vi "UHR-Fleezers Control (host) - 11.9b.vi"() -> ()   [LabVIEW 2014] (continued)
                  n310 = And(x=w552, y=w549) -> (x .and. y?=w551:bool)
                  n311 = case "Only if were fishing and now formed tether" shown="True" w551 {
                    tunnel: w550 -> [w554 w569]
                    tunnel: [w553 w568] -> w548
                    tunnel: w547 -> [_ w564]
                    frame False {
                      n312 = local read "Fish"() -> (w553:bool)
                      n313 = case shown="False" w553 {
                        tunnel: w554 -> [w555 _]
                        frame False {
                          n314 = property on="BD 1 Frequency 1 (MHz)" class="DigNum (strict)"("Val(Sgnl)"=w555) -> ()  [unwired: 2 in, 2 out]
                        }
                        frame True {
                        }
                      }
                    }
                    frame True {
                      w568 = FALSE ("Fish for Tether")
                      n315 = call <vilib>:"Beep.vi"() -> ()  [unwired: 3 in, 9 out]
                      n316 = Number To Decimal String(number=w564, width (-)=i16 1) -> (decimal integer string=w562:string)
                      n317 = Concatenate Strings("Formed tether in ", w562, " attempt(s)." ("string")) -> (w559:string)
                      n318 = local read "Messages"() -> (w566:string)
                      n319 = local write "Fish"(w568) -> ()
                      n320 = call "Update messages.vi"("Message to add"=w559, "Old message string"=w566) -> ("New message string"=w565:string)
                      n321 = local write "Messages"(w565) -> ()
                      n322 = Get Date/Time In Seconds() -> (seconds since 1Jan1904=→"Time tether formed":timestamp)
                      n323 = local read "Flow ON\nduring cal?"() -> (w556:bool)
                      n324 = property on="Sample Channel\nFlow" class="Bool (strict)"("Val(Sgnl)"=w556) -> (error out=w557:errorcluster)  [unwired: 2 in, 1 out]
                      n325 = case shown="\"2\", \"3\", \"4\", \"5\", \"6\"" "Then..." {
                        selector: "Then..." -> [_ w572 _ _]
                        tunnel: w569 -> [w571 _ _ _]
                        tunnel: w557 -> [_ _ _ _]
                        frame "1", Default {
                          n326 = property on="BD 1 Frequency 1 (MHz)" class="DigNum (strict)"("Val(Sgnl)"=w571) -> ()  [unwired: 2 in, 2 out]
                        }
                        frame "2", "3", "4", "5", "6" {
                          n327 = flat-sequence {
                            tunnel: w572 -> [w578]
                            frame #0 {
                              n328 = local read "Flow ON\nduring cal?"() -> (w573:bool)
                              n329 = property on="Sample Channel\nFlow" class="Bool (strict)"("Val(Sgnl)"=w573) -> ()  [unwired: 2 in, 2 out]
                              n330 = property on="Trap D (MHz)" class="DigNum (strict)"("Val(Sgnl)"="Move to D 1 (MHz)") -> ()  [unwired: 2 in, 2 out]
                            }
                            frame #1 {
                              n331 = local read "Wait Before Save (s)"() -> (w575:u32)
                              n332 = Multiply(x=u32 1000 ("milliseconds to wait"), y=w575) -> (x*y=w577:u32)
                              n333 = Wait (ms)(milliseconds to wait=w577) -> ()  [unwired: 1 out]
                            }
                            frame #2 {
                              n334 = case shown="\"5\", \"6\"" w578 {
                                selector: w578 -> [w581 w591 _]
                                frame "3", "4" {
                                n335 = flat-sequence {
                                tunnel: w581 -> [w582]
                                tunnel: [w582] -> w579
                                tunnel: [w584] -> w580
                                tunnel: w579 -> [w584]
                                tunnel: w580 -> [w588]
                                frame #0 {
                                n336 = property on="Green ON/Interlacing" class="Bool (strict)"("Val(Sgnl)"=TRUE ("Value (Signaling)")) -> ()  [unwired: 2 in, 2 out]
                                }
                                frame #1 {
                                n337 = Multiply(x="Wait Before Save (s)", y=u32 1000 ("x")) -> (x*y=w586:u32)
                                n338 = Wait (ms)(milliseconds to wait=w586) -> ()  [unwired: 1 out]
                                }
                                frame #2 {
                                n339 = property on="Start Saving" class="Bool (strict)"("Value"=TRUE ("Start Saving")) -> ()  [unwired: 2 in, 2 out]
                                n340 = case shown="\"4\"" w588 {
                                frame Default {
                                }
                                frame "4" {
                                n341 = property on="Fl. Triggered..." class="Bool (strict)"("Val(Sgnl)"=TRUE ("Value (Signaling)")) -> ()  [unwired: 2 in, 2 out]
                                }
                                }
                                }
                                }
                                }
                                frame "5", "6" {
                                n342 = stacked-sequence {
                                tunnel: w591 -> [_ _ _ _ _ _ w603]
                                frame #0 {
                                n343 = Replace Array Subset(array=u32[] [0] ("Index Values"), new element="Raster Set\nUpon Tether", index=0) -> (w592:u32[])
                                n344 = property on="Saved AOD Raster Scan Parameter Sets" class="Arr (strict)"("Index Values"=w592) -> ()  [unwired: 2 in, 2 out]
                                }
                                frame #1 {
                                n345 = Wait (ms)(milliseconds to wait=u32 500) -> ()  [unwired: 1 out]
                                }
                                frame #2 {
                                n346 = property on="Load parameters" class="Bool (strict)"("Val(Sgnl)"=TRUE ("Value (Signaling)")) -> ()  [unwired: 2 in, 2 out]
                                n347 = case shown="True" "Green ON during\nraster?" {
                                frame False {
                                }
                                frame True {
                                n348 = property on="Green ON/Interlacing" class="Bool (strict)"("Val(Sgnl)"=TRUE ("Value (Signaling)")) -> ()  [unwired: 2 in, 2 out]
                                }
                                }
                                }
                                frame #3 {
                                n349 = Wait (ms)(milliseconds to wait=u32 500) -> ()  [unwired: 1 out]
                                }
                                frame #4 {
                                n350 = property on="Trap Raster Scan" class="Bool (strict)"("Val(Sgnl)"=TRUE ("Value (Signaling)")) -> ()  [unwired: 2 in, 2 out]
                                }
                                frame #5 {
                                n351 = Wait (ms)(milliseconds to wait=u32 2000) -> ()  [unwired: 1 out]
                                }
                                frame #6 {
                                n352 = flat-sequence {
                                tunnel: w603 -> [w610]
                                frame #0 {
                                n353 = while {
                                stop <- w606 stop-if-true
                                n354 = local read "Raster Scanning..."() -> (w605:bool)
                                n355 = local read "Saving..."() -> (w608:bool)
                                n356 = Wait (ms)(milliseconds to wait=u32 100) -> ()  [unwired: 1 out]
                                n357 = Not(x=w608) -> (.not. x?=w607:bool)
                                n358 = Not(x=w605) -> (.not. x?=w604:bool)
                                n359 = And(x=w607, y=w604) -> (x .and. y?=w606:bool)
                                }
                                }
                                frame #1 {
                                n360 = local read "Tether"() -> (w611:bool)
                                n361 = case shown="True" w611 {
                                tunnel: w610 -> [_ w613]
                                frame False {
                                n362 = property on="Fish" class="Bool (strict)"("Val(Sgnl)"="Fish again after \nraster break?") -> ()  [unwired: 2 in, 2 out]
                                }
                                frame True {
                                n363 = stacked-sequence {
                                tunnel: w613 -> [_ w617 _ _ _ _ _ _]
                                frame #0 {
                                n364 = property on="Trap D (MHz)" class="DigNum (strict)"("Val(Sgnl)"="Move to D 2 (MHz)") -> ()  [unwired: 2 in, 2 out]
                                n365 = case shown="True" "Flow ON after\ntether testing?" {
                                frame False {
                                }
                                frame True {
                                n366 = property on="Sample Channel\nFlow" class="Bool (strict)"("Val(Sgnl)"=TRUE ("Value (Signaling)")) -> ()  [unwired: 2 in, 2 out]
                                }
                                }
                                }
                                frame #1 {
                                n367 = flat-sequence {
                                tunnel: w617 -> [w618]
                                frame #0 {
                                n368 = case shown="\"6\"" w618 {
                                frame Default {
                                }
                                frame "6" {
                                n369 = flat-sequence {
                                frame #0 {
                                n370 = Wait (ms)(milliseconds to wait=u32 500) -> ()  [unwired: 1 out]
                                }
                                frame #1 {
                                n371 = property on="Green ON/Interlacing" class="Bool (strict)"("Val(Sgnl)"=TRUE ("Green Laser ON/Interlacing")) -> ()  [unwired: 2 in, 2 out]
                                }
                                }
                                }
                                }
                                }
                                frame #1 {
                                n372 = case shown="True" "Save at end (5, 6)" {
                                selector: "Save at end (5, 6)" -> [_ w622]
                                frame False {
                                }
                                frame True {
                                n373 = flat-sequence {
                                tunnel: w622 -> [w624]
                                frame #0 {
                                n374 = Wait (ms)(milliseconds to wait=u32 500) -> ()  [unwired: 1 out]
                                }
                                frame #1 {
                                n375 = local write "Start Saving"(w624) -> ()
                                }
                                }
                                }
                                }
                                }
                                }
                                }
                                frame #2 {
                                n376 = local read "Bead Sep. Int. Time (s)"() -> (w627:dbl)
                                n377 = Multiply(x=w627, y=1000.0) -> (x*y=w626:dbl)
                                n378 = Wait (ms)(milliseconds to wait=w626) -> ()  [unwired: 1 out]
                                }
                                frame #3 {
                                n379 = property on="Remove Offset" class="Bool (strict)"("Val(Sgnl)"=TRUE ("Value (Signaling)")) -> ()  [unwired: 2 in, 2 out]
                                }
                                frame #4 {
                                n380 = property on="Read FX file" class="Bool (strict)"("Val(Sgnl)"=TRUE ("Value (Signaling)")) -> ()  [unwired: 2 in, 2 out]
                                }
                                frame #5 {
                                n381 = Wait (ms)(milliseconds to wait=u32 300) -> ()  [unwired: 1 out]
                                }
                                frame #6 {
                                n382 = local read "Bad fit error"() -> (w636:dbl)
                                n383 = local read "Fit offset"() -> (w639:dbl)
                                n384 = Greater Or Equal?(x=w636, y="Bad fit thresh") -> (x >= y?=→"Bad fit":bool)
                                n385 = Greater Or Equal?(x=w639, y="Fit offset thresh") -> (x >= y?=→"Multiple tether":bool)
                                n386 = local read "Hyst. error"() -> (w633:dbl)
                                n387 = Greater Or Equal?(x=w633, y="Hysteresis thresh") -> (x >= y?=→"Hysteresis":bool)
                                }
                                frame #7 {
                                w644 = 0
                                n388 = local read "Bad fit error"() -> (w646:dbl)
                                n389 = local read "Hyst. error"() -> (w645:dbl)
                                n390 = local read "Fit offset"() -> (w647:dbl)
                                n391 = local read "Multiple tether"() -> (w653:bool)
                                n392 = local read "Hysteresis"() -> (w651:bool)
                                n393 = local read "Bad fit"() -> (w652:bool)
                                n394 = Not(x=w651) -> (.not. x?=w643:bool)
                                n395 = Not(x=w652) -> (.not. x?=w649:bool)
                                n396 = Greater?(x=w647, y=w644) -> (0:w642:bool)
                                n397 = Greater?(x=w646, y=w644) -> (0:w641:bool)
                                n398 = Greater?(x=w645, y=w644) -> (0:w640:bool)
                                n399 = Not(x=w653) -> (.not. x?=w650:bool)
                                n400 = Compound Arithmetic op=AND(w650, w649, w643, w642, w641, w640) -> (w648:bool)
                                "Good tether" <- w648
                                n401 = case shown="True" w648 {
                                frame False {
                                }
                                frame True {
                                n402 = call <vilib>:"Beep.vi"("use system alert? (T)"=FALSE, "duration (msec)"=u32 200, "frequency (Hz)"=u32 2000) -> ()  [unwired: 9 in]
                                }
                                }
                                }
                                }
                                }
                                }
                                }
                                }
                                }
                                }
                                }
                                frame "2", Default {
                                }
                              }
                            }
                            frame #3 {
                              n403 = local read "Multiple tether"() -> (w659:bool)
                              n404 = And(x="Break multiple", y=w659) -> (x .and. y?=w657:bool)
                              n405 = case shown="True" w657 {
                                frame False {
                                }
                                frame True {
                                n406 = stacked-sequence {
                                frame #0 {
                                n407 = property on="Trap D (MHz)" class="DigNum (strict)"("Val(Sgnl)"="Trap D to \nbreak (MHz)") -> ()  [unwired: 2 in, 2 out]
                                }
                                frame #1 {
                                n408 = case shown="True" "Fish after\nmultiple break" {
                                frame False {
                                }
                                frame True {
                                n409 = while {
                                stop <- w664 stop-if-true
                                n410 = local read "Multiple tether"() -> (w666:bool)
                                n411 = local read "Fish"() -> (w663:bool)
                                n412 = local read "Stop All"() -> (w662:bool)
                                n413 = Wait (ms)(milliseconds to wait=u32 100) -> ()  [unwired: 1 out]
                                n414 = Not(x=w666) -> (.not. x?=w665:bool)
                                n415 = Compound Arithmetic op=OR(w662, w665, w663) -> (w664:bool)
                                }
                                }
                                }
                                }
                                frame #2 {
                                n416 = local read "Fish after\nmultiple break"() -> (w671:bool)
                                n417 = local read "Stage Moving"() -> (w670:bool)
                                n418 = Not(x=w670) -> (.not. x?=w668:bool)
                                n419 = And(x=w671, y=w668) -> (x .and. y?=w669:bool)
                                n420 = property on="Fish" class="Bool (strict)"("Val(Sgnl)"=w669) -> ()  [unwired: 2 in, 2 out]
                                }
                                }
                                }
                              }
                            }
                            frame #4 {
                              n421 = local read "Bad fit"() -> (w673:bool)
                              n422 = And(x="Break bad fit", y=w673) -> (x .and. y?=w672:bool)
                              n423 = case shown="True" w672 {
                                frame False {
                                }
                                frame True {
                                n424 = stacked-sequence {
                                frame #0 {
                                n425 = local read "Trap D to \nbreak (MHz)"() -> (w675:dbl)
                                n426 = property on="Trap D (MHz)" class="DigNum (strict)"("Val(Sgnl)"=w675) -> ()  [unwired: 2 in, 2 out]
                                }
                                frame #1 {
                                n427 = case shown="True" "Fish after\nbad fit break?" {
                                frame False {
                                }
                                frame True {
                                n428 = while {
                                stop <- w679 stop-if-true
                                n429 = local read "Stop All"() -> (w677:bool)
                                n430 = local read "Bad fit"() -> (w678:bool)
                                n431 = local read "Fish"() -> (w680:bool)
                                n432 = Not(x=w678) -> (.not. x?=w681:bool)
                                n433 = Wait (ms)(milliseconds to wait=u32 100) -> ()  [unwired: 1 out]
                                n434 = Compound Arithmetic op=OR(w677, w681, w680) -> (w679:bool)
                                }
                                }
                                }
                                }
                                frame #2 {
                                n435 = local read "Fish after\nbad fit break?"() -> (w683:bool)
                                n436 = local read "Stage Moving"() -> (w686:bool)
                                n437 = Not(x=w686) -> (.not. x?=w685:bool)
                                n438 = And(x=w683, y=w685) -> (x .and. y?=w684:bool)
                                n439 = property on="Fish" class="Bool (strict)"("Val(Sgnl)"=w684) -> ()  [unwired: 2 in, 2 out]
                                }
                                }
                                }
                              }
                            }
                            frame #5 {
                              n440 = local read "Hysteresis"() -> (w688:bool)
                              n441 = And(x="Break hyst", y=w688) -> (x .and. y?=w687:bool)
                              n442 = case shown="True" w687 {
                                frame False {
                                }
                                frame True {
                                n443 = stacked-sequence {
                                frame #0 {
                                n444 = local read "Trap D to \nbreak (MHz)"() -> (w690:dbl)
                                n445 = property on="Trap D (MHz)" class="DigNum (strict)"("Val(Sgnl)"=w690) -> ()  [unwired: 2 in, 2 out]
                                }
                                frame #1 {
                                n446 = case shown="True" "Fish ater hyst?" {
                                frame False {
                                }
                                frame True {
                                n447 = while {
                                stop <- w696 stop-if-true
                                n448 = local read "Hysteresis"() -> (w695:bool)
                                n449 = local read "Stop All"() -> (w692:bool)
                                n450 = local read "Fish"() -> (w693:bool)
                                n451 = Wait (ms)(milliseconds to wait=u32 100) -> ()  [unwired: 1 out]
                                n452 = Not(x=w695) -> (.not. x?=w694:bool)
                                n453 = Compound Arithmetic op=OR(w692, w694, w693) -> (w696:bool)
                                }
                                }
                                }
                                }
                                frame #2 {
                                n454 = local read "Fish ater hyst?"() -> (w701:bool)
                                n455 = local read "Stage Moving"() -> (w700:bool)
                                n456 = Not(x=w700) -> (.not. x?=w699:bool)
                                n457 = And(x=w701, y=w699) -> (x .and. y?=w698:bool)
                                n458 = property on="Fish" class="Bool (strict)"("Val(Sgnl)"=w698) -> ()  [unwired: 2 in, 2 out]
                                }
                                }
                                }
                              }
                            }
                            frame #6 {
                              n459 = local read "Good tether"() -> (w702:bool)
                              n460 = case shown="True" w702 {
                                frame False {
                                }
                                frame True {
                                n461 = case shown="\"1\"" "If good, then:" {
                                frame "0", Default {
                                }
                                frame "1" {
                                n462 = property on="Force FB Script" class="Bool (strict)"("Val(Sgnl)"=TRUE ("Value (Signaling)")) -> ()  [unwired: 2 in, 2 out]
                                }
                                }
                                }
                              }
                            }
                          }
                        }
                        frame "7" {
                          n463 = property on="Force FB Script" class="Bool (strict)"("Val(Sgnl)"=TRUE ("Value (Signaling)")) -> ()  [unwired: 2 in, 2 out]
                        }
                        frame "8" {
                          n464 = property on="Fixed Traps Script" class="Bool (strict)"("Val(Sgnl)"=TRUE ("Value (Signaling)")) -> ()  [unwired: 2 in, 2 out]
                        }
                      }
                      "Tether" <- "Tether Alarm?"
                    }
                  }
                }
                frame #2 {
                  n465 = local read "Oscillate Set 1"() -> (w712:bool)
                  n466 = local read "Stop All"() -> (w710:bool)
                  n467 = Or(x=w712, y=w707) -> (x .or. y?=w709:bool)
                  n468 = Not(x=w709) -> (.not. x?=w711:bool)
                  n469 = Compound Arithmetic op=OR(w710, w711) -> (w708:bool)
                }
              }
              n470 = node-c288() -> ()  [unwired: 2 out]
            }
            n471 = node-c288(w462) -> ()  [unwired: 1 out]
          }
        }
      }
      event "Fl. Triggered...": Value Change {
        n472 = event-data() -> ()  [unwired: 7 out]
        n473 = case shown="True" "Fl. Triggered..." {
          frame False {
          }
          frame True {
            n474 = node-c288() -> (w723:T21)  [unwired: 4 out]
            n475 = timed-loop {
              timing: w723 -> [_]
              timing-out: [_] -> w722
              tunnel: "Action" -> [w731]
              shift-right: [w728] -> _
              shift-left: u8 255 -> [w730]
              shift-right: [w725] -> _
              shift-left: 255 -> [w727]
              stop <- w724 stop-if-true
              # "Reset confocal spot"
              n476 = node-c288() -> ()  [unwired: 2 out]
              n477 = flat-sequence {
                tunnel: w731 -> [w751]
                tunnel: w730 -> [w750]
                tunnel: [w749] -> w729
                tunnel: w727 -> [w736]
                tunnel: [w735] -> w726
                tunnel: [w1135] -> w724
                tunnel: w729 -> [w1134]
                tunnel: [w1134] -> w728
                tunnel: [w1133] -> w725
                tunnel: w726 -> [w1133]
                frame #0 {
                  n478 = local read "Delta Fl. 2"() -> (w748:dbl)
                  n479 = local read "Delta Fl. 1"() -> (w743:dbl)
                  n480 = Multiply(x="Fl. D Thresh. (kHz)", y=1000.0) -> (x*y=w738:dbl)
                  n481 = Select(t=w743, s="APD to Watch", f=w748) -> (s? t:f=w739:dbl)
                  n482 = Greater?(x=w739, y=w738) -> (0:w744:bool)
                  n483 = Or(x="Force Yank", y=w744) -> (x .or. y?=w742:bool)
                  n484 = And(x=w742, y="Yank when?") -> (x .and. y?=w740:bool)
                  n485 = case shown="False" w740 {
                    tunnel: w751 -> [w754 w957]
                    tunnel: w750 -> [w756 w953]
                    tunnel: [w756 w951] -> w749
                    tunnel: w739 -> [w762 _]
                    tunnel: w738 -> [w761 _]
                    tunnel: "Force Yank" -> [w759 _]
                    tunnel: w736 -> [w758 w950]
                    tunnel: [w757 w950] -> w735
                    frame False {
                      n486 = Negate(x=w761) -> (-x=w753:dbl)
                      n487 = local write "Fl. High"(TRUE ("Fl. High")) -> ()
                      n488 = Less?(x=w762, y=w753) -> (x < y?=w760:bool)
                      n489 = Or(x=w759, y=w760) -> (x .or. y?=w755:bool)
                      n490 = case shown="True" w755 {
                        tunnel: w758 -> [w763 w773]
                        tunnel: [w763 w772] -> w757
                        tunnel: w754 -> [_ w771]
                        frame False {
                        }
                        frame True {
                          n491 = flat-sequence {
                            tunnel: w773 -> [w779]
                            tunnel: w771 -> [w776]
                            tunnel: [w778] -> w770
                            tunnel: [w777] -> w769
                            tunnel: [w776] -> w768
                            tunnel: w767 -> [w775]
                            tunnel: [w775] -> w766
                            tunnel: w765 -> [w774]
                            tunnel: [w774] -> w764
                            tunnel: [w851] -> w772
                            tunnel: w770 -> [w851]
                            tunnel: w769 -> [w850]
                            tunnel: w768 -> [w849]
                            tunnel: w766 -> [w848]
                            tunnel: w764 -> [w847]
                            frame #0 {
                              n492 = call <vilib>:"Beep.vi"() -> ()  [unwired: 12 in]
                              n493 = local write "Waiting"(FALSE ("Waiting")) -> ()
                              n494 = Increment(x=w779) -> (x+1=w778:i32)
                              n495 = case shown="\"Yank\"" w776 {
                                tunnel: w778 -> [_ w784 _]
                                frame "Alarm", Default {
                                }
                                frame "Yank" {
                                n496 = flat-sequence {
                                tunnel: w784 -> [w787]
                                tunnel: [w786] -> w783
                                tunnel: [w785] -> w782
                                tunnel: w783 -> [w797]
                                tunnel: w782 -> [w798]
                                frame #0 {
                                n497 = local read "Yank Delay (s)"() -> (w790:dbl)
                                n498 = local read "N Array El"() -> (w785:u8)
                                n499 = Quotient & Remainder(x=w787, y=w785) -> (x-y*floor(x/y)=w786:i32)  [unwired: 1 out]
                                n500 = Multiply(x=w790, y=1000.0) -> (x*y=w788:dbl)
                                n501 = Wait (ms)(milliseconds to wait=w788) -> ()  [unwired: 1 out]
                                }
                                frame #1 {
                                n502 = local read "Yank to which?"() -> (w792:bool)
                                n503 = local read "Random Choice"() -> (w802:bool)
                                n504 = local read "Yank to Trap D (MHz)"() -> (w795:dbl[])
                                n505 = local read "Yank to SP"() -> (w796:dbl[])
                                n506 = Random Number (0-1)() -> (number: 0 to 1=w801:dbl)
                                n507 = Multiply(x=w798, y=w801) -> (x*y=w800:dbl)
                                n508 = Round Toward -Infinity(1:w800) -> (0:w799:dbl)
                                n509 = Select(t=w799, s=w802, f=w797) -> (s? t:f=w793:dbl)
                                n510 = Select(t=w795, s=w792, f=w796) -> (s? t:f=w794:dbl[])
                                n511 = Index Array(array=w794, index=w793) -> (element=w791:dbl)
                                n512 = case shown="False" w792 {
                                tunnel: w791 -> [w803 w831]
                                frame False {
                                n513 = flat-sequence {
                                tunnel: w803 -> [w804]
                                frame #0 {
                                n514 = property on="Trap Pos FB SP" class="DigNum (strict)"("Val(Sgnl)"=w804) -> ()  [unwired: 2 in, 2 out]
                                }
                                frame #1 {
                                n515 = Wait (ms)(milliseconds to wait=u32 700) -> ()  [unwired: 1 out]
                                }
                                frame #2 {
                                n516 = local read "Action (%)"() -> (w809:dbl)
                                n517 = Absolute Value(x=w809) -> (abs(x)=w808:dbl)
                                n518 = Greater?(x=w808, y=70.0) -> (0:w806:bool)
                                n519 = property on="Remove Action Offset" class="Bool (strict)"("Val(Sgnl)"=w806) -> ()  [unwired: 2 in, 2 out]
                                }
                                frame #3 {
                                n520 = for {
                                N: 4 -> [_]
                                n521 = flat-sequence {
                                frame #0 {
                                n522 = Wait (ms)(milliseconds to wait=u32 500) -> ()  [unwired: 1 out]
                                }
                                frame #1 {
                                n523 = local read "Action (%)"() -> (w815:dbl)
                                n524 = Absolute Value(x=w815) -> (abs(x)=w814:dbl)
                                n525 = Greater?(x=w814, y=70.0) -> (0:w812:bool)
                                n526 = property on="Remove Action Offset" class="Bool (strict)"("Val(Sgnl)"=w812) -> ()  [unwired: 2 in, 2 out]
                                }
                                }
                                }
                                }
                                frame #4 {
                                n527 = Wait (ms)(milliseconds to wait=u32 500) -> ()  [unwired: 1 out]
                                }
                                frame #5 {
                                n528 = local read "Mean"() -> (w823:dbl)
                                n529 = Greater?(x=w823, y=11.0) -> (0:w817:bool)
                                n530 = Not(x=w817) -> (.not. x?=w818:bool)
                                n531 = And(x=w818, y="Shift confocal") -> (x .and. y?=w820:bool)
                                n532 = And(x=w817, y="Shift confocal") -> (x .and. y?=w821:bool)
                                n533 = case shown="True" w821 {
                                frame False {
                                }
                                frame True {
                                n534 = local read "Confocal Y 2 (V)"() -> (w827:dbl)
                                n535 = local read "Confocal X 2 (V)"() -> (w826:dbl)
                                n536 = property on="AO1" class="Slide (strict)"("Val(Sgnl)"=w827) -> ()  [unwired: 2 in, 2 out]
                                n537 = property on="AO2" class="Slide (strict)"("Val(Sgnl)"=w826) -> ()  [unwired: 2 in, 2 out]
                                }
                                }
                                n538 = case shown="True" w820 {
                                frame False {
                                }
                                frame True {
                                n539 = local read "Confocal Y 1 (V)"() -> (w825:dbl)
                                n540 = local read "Confocal X 1 (V)"() -> (w824:dbl)
                                n541 = property on="AO1" class="Slide (strict)"("Val(Sgnl)"=w825) -> ()  [unwired: 2 in, 2 out]
                                n542 = property on="AO2" class="Slide (strict)"("Val(Sgnl)"=w824) -> ()  [unwired: 2 in, 2 out]
                                }
                                }
                                }
                                frame #6 {
                                n543 = Wait (ms)(milliseconds to wait=u32 1500) -> ()  [unwired: 1 out]
                                }
                                frame #7 {
                                n544 = property on="Rem fb disp offset" class="Bool (strict)"("Val(Sgnl)"=TRUE ("Value (Signaling)")) -> ()  [unwired: 2 in, 2 out]
                                n545 = property on="Remove Offset" class="Bool (strict)"("Val(Sgnl)"=TRUE ("Value (Signaling)")) -> ()  [unwired: 2 in, 2 out]
                                }
                                }
                                }
                                frame True {
                                n546 = flat-sequence {
                                tunnel: w831 -> [w832]
                                frame #0 {
                                n547 = property on="Trap D (MHz)" class="DigNum (strict)"("Val(Sgnl)"=w832) -> ()  [unwired: 2 in, 2 out]
                                }
                                frame #1 {
                                n548 = Wait (ms)(milliseconds to wait=u32 500) -> ()  [unwired: 1 out]
                                }
                                frame #2 {
                                n549 = local read "Shift confocal"() -> (w838:bool)
                                n550 = local read "Mean"() -> (w840:dbl)
                                n551 = Greater?(x=w840, y=11.0) -> (0:w837:bool)
                                n552 = Not(x=w837) -> (.not. x?=w836:bool)
                                n553 = And(x=w836, y=w838) -> (x .and. y?=w834:bool)
                                n554 = And(x=w837, y=w838) -> (x .and. y?=w835:bool)
                                n555 = case shown="True" w835 {
                                frame False {
                                }
                                frame True {
                                n556 = local read "Confocal Y 2 (V)"() -> (w844:dbl)
                                n557 = local read "Confocal X 2 (V)"() -> (w843:dbl)
                                n558 = property on="AO2" class="Slide (strict)"("Val(Sgnl)"=w843) -> ()  [unwired: 2 in, 2 out]
                                n559 = property on="AO1" class="Slide (strict)"("Val(Sgnl)"=w844) -> ()  [unwired: 2 in, 2 out]
                                }
                                }
                                n560 = case shown="True" w834 {
                                frame False {
                                }
                                frame True {
                                n561 = local read "Confocal X 1 (V)"() -> (w841:dbl)
                                n562 = local read "Confocal Y 1 (V)"() -> (w842:dbl)
                                n563 = property on="AO2" class="Slide (strict)"("Val(Sgnl)"=w841) -> ()  [unwired: 2 in, 2 out]
                                n564 = property on="AO1" class="Slide (strict)"("Val(Sgnl)"=w842) -> ()  [unwired: 2 in, 2 out]
                                }
                                }
                                }
                                }
                                }
                                }
                                }
                                }
                                }
                                frame "Image" {
                                n565 = property on="Confocal\nImage" class="Bool (strict)"("Val(Sgnl)"=TRUE ("Value (Signaling)")) -> ()  [unwired: 2 in, 2 out]
                                }
                              }
                              n566 = local write "Fl. High"(FALSE ("Fl. High")) -> ()
                              n567 = local read "Time (s)"() -> (w777:dbl)
                            }
                            frame #1 {
                              n568 = case shown="True" "Auto F Reset" {
                                tunnel: w850 -> [_ w855]
                                tunnel: w849 -> [_ w854]
                                tunnel: w848 -> [_ w853]
                                tunnel: w847 -> [_ w852]
                                frame False {
                                }
                                frame True {
                                n569 = node-c288() -> (w857:T21)  [unwired: 4 in]
                                n570 = timed-loop {
                                timing: w857 -> [_]
                                timing-out: [_] -> w856
                                tunnel: w855 -> [w862]
                                tunnel: w854 -> [w861]
                                tunnel: w853 -> [w860]
                                tunnel: w852 -> [w859]
                                stop <- w858 stop-if-true
                                n571 = node-c288() -> ()  [unwired: 1 in, 1 out]
                                n572 = local read "APD to Watch"() -> (w872:bool)
                                n573 = local read "Fl. D Thresh. (kHz)"() -> (w871:dbl)
                                n574 = local read "Delta Fl. 1"() -> (w873:dbl)
                                n575 = local read "Delta Fl. 2"() -> (w874:dbl)
                                n576 = local read "Fl. Triggered..."() -> (w865:bool)
                                n577 = local read "Stop All"() -> (w866:bool)
                                n578 = local read "Reset Force"() -> (w864:bool)
                                n579 = Multiply(x=w871, y=1000.0) -> (x*y=w869:dbl)
                                n580 = Not(x=w865) -> (.not. x?=w863:bool)
                                n581 = Select(t=w873, s=w872, f=w874) -> (s? t:f=w868:dbl)
                                n582 = Greater?(x=w868, y=w869) -> (0:w867:bool)
                                n583 = Compound Arithmetic op=OR(w867, w866, w863, w864) -> (w858:bool)
                                n584 = case shown="True" w858 {
                                tunnel: w862 -> [_ w878]
                                tunnel: w861 -> [_ w882]
                                tunnel: w860 -> [_ w881]
                                tunnel: w859 -> [_ w880]
                                frame False {
                                }
                                frame True {
                                n585 = case shown="\"Yank\"" w882 {
                                tunnel: w881 -> [_ w892]
                                tunnel: w880 -> [_ w890]
                                frame "Image", Default {
                                }
                                frame "Yank" {
                                n586 = flat-sequence {
                                tunnel: [w895] -> w893
                                tunnel: w892 -> [w895]
                                tunnel: [w894] -> w891
                                tunnel: w890 -> [w894]
                                tunnel: w893 -> [w901]
                                tunnel: w891 -> [w899]
                                frame #0 {
                                n587 = local read "Yank Delay (s)"() -> (w898:dbl)
                                n588 = Multiply(x=w898, y=1000.0) -> (x*y=w896:dbl)
                                n589 = Wait (ms)(milliseconds to wait=w896) -> ()  [unwired: 1 out]
                                }
                                frame #1 {
                                n590 = local read "Yank to which?"() -> (w900:bool)
                                n591 = case shown="False" w900 {
                                tunnel: w901 -> [_ w930]
                                tunnel: w899 -> [w902 _]
                                frame False {
                                n592 = flat-sequence {
                                tunnel: w902 -> [w903]
                                frame #0 {
                                n593 = property on="Trap Pos FB SP" class="DigNum (strict)"("Val(Sgnl)"=w903) -> ()  [unwired: 2 in, 2 out]
                                }
                                frame #1 {
                                n594 = Wait (ms)(milliseconds to wait=u32 700) -> ()  [unwired: 1 out]
                                }
                                frame #2 {
                                n595 = local read "Action (%)"() -> (w908:dbl)
                                n596 = Absolute Value(x=w908) -> (abs(x)=w907:dbl)
                                n597 = Greater?(x=w907, y=70.0) -> (0:w905:bool)
                                n598 = property on="Remove Action Offset" class="Bool (strict)"("Val(Sgnl)"=w905) -> ()  [unwired: 2 in, 2 out]
                                }
                                frame #3 {
                                n599 = for {
                                N: 4 -> [_]
                                n600 = flat-sequence {
                                frame #0 {
                                n601 = Wait (ms)(milliseconds to wait=u32 500) -> ()  [unwired: 1 out]
                                }
                                frame #1 {
                                n602 = local read "Action (%)"() -> (w914:dbl)
                                n603 = Absolute Value(x=w914) -> (abs(x)=w913:dbl)
                                n604 = Greater?(x=w913, y=70.0) -> (0:w911:bool)
                                n605 = property on="Remove Action Offset" class="Bool (strict)"("Val(Sgnl)"=w911) -> ()  [unwired: 2 in, 2 out]
                                }
                                }
                                }
                                }
                                frame #4 {
                                n606 = Wait (ms)(milliseconds to wait=u32 500) -> ()  [unwired: 1 out]
                                }
                                frame #5 {
                                n607 = local read "Shift confocal"() -> (w919:bool)
                                n608 = local read "Mean"() -> (w922:dbl)
                                n609 = Greater?(x=w922, y=11.0) -> (0:w918:bool)
                                n610 = Not(x=w918) -> (.not. x?=w917:bool)
                                n611 = And(x=w918, y=w919) -> (x .and. y?=w920:bool)
                                n612 = And(x=w917, y=w919) -> (x .and. y?=w916:bool)
                                n613 = case shown="True" w920 {
                                frame False {
                                }
                                frame True {
                                n614 = local read "Confocal X 2 (V)"() -> (w925:dbl)
                                n615 = local read "Confocal Y 2 (V)"() -> (w926:dbl)
                                n616 = property on="AO2" class="Slide (strict)"("Val(Sgnl)"=w925) -> ()  [unwired: 2 in, 2 out]
                                n617 = property on="AO1" class="Slide (strict)"("Val(Sgnl)"=w926) -> ()  [unwired: 2 in, 2 out]
                                }
                                }
                                n618 = case shown="True" w916 {
                                frame False {
                                }
                                frame True {
                                n619 = local read "Confocal Y 1 (V)"() -> (w924:dbl)
                                n620 = local read "Confocal X 1 (V)"() -> (w923:dbl)
                                n621 = property on="AO1" class="Slide (strict)"("Val(Sgnl)"=w924) -> ()  [unwired: 2 in, 2 out]
                                n622 = property on="AO2" class="Slide (strict)"("Val(Sgnl)"=w923) -> ()  [unwired: 2 in, 2 out]
                                }
                                }
                                }
                                frame #6 {
                                n623 = Wait (ms)(milliseconds to wait=u32 1500) -> ()  [unwired: 1 out]
                                }
                                frame #7 {
                                n624 = property on="Remove Offset" class="Bool (strict)"("Val(Sgnl)"=TRUE ("Value (Signaling)")) -> ()  [unwired: 2 in, 2 out]
                                n625 = property on="Rem fb disp offset" class="Bool (strict)"("Val(Sgnl)"=TRUE ("Value (Signaling)")) -> ()  [unwired: 2 in, 2 out]
                                }
                                }
                                }
                                frame True {
                                n626 = flat-sequence {
                                tunnel: w930 -> [w931]
                                frame #0 {
                                n627 = property on="Trap D (MHz)" class="DigNum (strict)"("Val(Sgnl)"=w931) -> ()  [unwired: 2 in, 2 out]
                                }
                                frame #1 {
                                n628 = Wait (ms)(milliseconds to wait=u32 500) -> ()  [unwired: 1 out]
                                }
                                frame #2 {
                                n629 = local read "Shift confocal"() -> (w937:bool)
                                n630 = local read "Mean"() -> (w938:dbl)
                                n631 = Greater?(x=w938, y=11.0) -> (0:w936:bool)
                                n632 = And(x=w936, y=w937) -> (x .and. y?=w934:bool)
                                n633 = Not(x=w936) -> (.not. x?=w935:bool)
                                n634 = And(x=w935, y=w937) -> (x .and. y?=w933:bool)
                                n635 = case shown="True" w934 {
                                frame False {
                                }
                                frame True {
                                n636 = local read "Confocal Y 2 (V)"() -> (w943:dbl)
                                n637 = local read "Confocal X 2 (V)"() -> (w942:dbl)
                                n638 = property on="AO1" class="Slide (strict)"("Val(Sgnl)"=w943) -> ()  [unwired: 2 in, 2 out]
                                n639 = property on="AO2" class="Slide (strict)"("Val(Sgnl)"=w942) -> ()  [unwired: 2 in, 2 out]
                                }
                                }
                                n640 = case shown="True" w933 {
                                frame False {
                                }
                                frame True {
                                n641 = local read "Confocal Y 1 (V)"() -> (w941:dbl)
                                n642 = local read "Confocal X 1 (V)"() -> (w940:dbl)
                                n643 = property on="AO2" class="Slide (strict)"("Val(Sgnl)"=w940) -> ()  [unwired: 2 in, 2 out]
                                n644 = property on="AO1" class="Slide (strict)"("Val(Sgnl)"=w941) -> ()  [unwired: 2 in, 2 out]
                                }
                                }
                                }
                                }
                                }
                                }
                                }
                                }
                                }
                                }
                                n645 = local read "Time (s)"() -> (w877:dbl)
                                n646 = Subtract(x=w878, y=w877) -> (x-y=w889:dbl)
                                n647 = Number To Decimal String(number=w889, width (-)=i16 0) -> (decimal integer string=w887:string)
                                n648 = Concatenate Strings(w887, " s fluorescence event") -> (w884:string)
                                n649 = local read "Messages"() -> (w885:string)
                                n650 = local write "Duration (s)"(w889) -> ()
                                n651 = call "Update messages.vi"("Message to add"=w884, "Old message string"=w885) -> ("New message string"=w883:string)
                                n652 = local write "Messages"(w883) -> ()
                                n653 = call <vilib>:"Beep.vi"() -> ()  [unwired: 12 in]
                                n654 = local write "Reset Force"(FALSE ("Force Reset")) -> ()
                                n655 = local write "Fl. High"(TRUE ("Fl. High")) -> ()
                                n656 = local write "Waiting"(TRUE ("Waiting")) -> ()
                                }
                                }
                                n657 = node-c288() -> ()  [unwired: 1 in, 1 out]
                                }
                                n658 = node-c288(w856) -> ()  [unwired: 1 out]
                                }
                              }
                            }
                          }
                          n659 = local read "Trap Pos FB SP"() -> (w765:fxp<+/-,16,1>)
                          n660 = local read "Trap D (MHz)"() -> (w767:dbl)
                        }
                      }
                    }
                    frame True {
                      n661 = flat-sequence {
                        tunnel: w954 -> [w964]
                        tunnel: [w964] -> w958
                        tunnel: w957 -> [w963]
                        tunnel: [w963] -> w956
                        tunnel: [w962] -> w955
                        tunnel: w953 -> [w961]
                        tunnel: [w960] -> w952
                        tunnel: w949 -> [w959]
                        tunnel: [w959] -> w948
                        tunnel: w958 -> [w1036]
                        tunnel: w956 -> [w1035]
                        tunnel: w955 -> [w1034]
                        tunnel: w952 -> [w1033]
                        tunnel: w948 -> [w1032]
                        tunnel: [w1033] -> w951
                        frame #0 {
                          n662 = call <vilib>:"Beep.vi"() -> ()  [unwired: 3 in, 9 out]
                          n663 = local write "Waiting"(FALSE ("Waiting")) -> ()
                          n664 = Increment(x=w961) -> (x+1=w960:u8)
                          n665 = case shown="\"Image\"" w963 {
                            tunnel: w960 -> [_ _ w970 _]
                            frame "Image" {
                              n666 = property on="Confocal\nImage" class="Bool (strict)"("Val(Sgnl)"=TRUE ("Value (Signaling)")) -> ()  [unwired: 2 in, 2 out]
                            }
                            frame "Alarm", Default {
                            }
                            frame "Yank" {
                              n667 = flat-sequence {
                                tunnel: w970 -> [w973]
                                tunnel: [w972] -> w969
                                tunnel: ["N Array El"] -> w968
                                tunnel: w969 -> [w987]
                                tunnel: w968 -> [w983]
                                frame #0 {
                                n668 = Multiply(x="Yank Delay (s)", y=1000.0) -> (x*y=w976:dbl)
                                n669 = Quotient & Remainder(x=w973, y="N Array El") -> (x-y*floor(x/y)=w972:u8)  [unwired: 1 out]
                                n670 = Wait (ms)(milliseconds to wait=w976) -> ()  [unwired: 1 out]
                                }
                                frame #1 {
                                n671 = Random Number (0-1)() -> (number: 0 to 1=w984:dbl)
